vi "CANShark_SetBitrate.vi"(8 "Data Bitrate":i32, 9 "Nominal Bitrate":i32, 10 "Device Handler":i64, 11 "error in (no error)":errorcluster) -> (2 "CanFD Bitrate":u8, 3 "error out":errorcluster)   [LabVIEW 2026]
uses:
  x64/Release/CanSharkApi_Dll1.dll
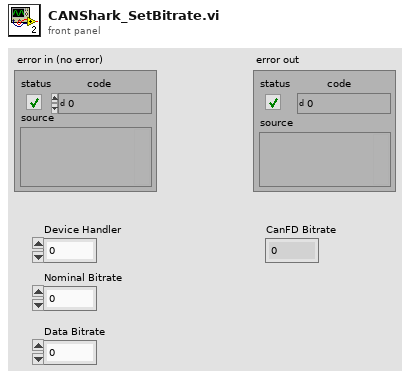
[diagram p1: front panel]
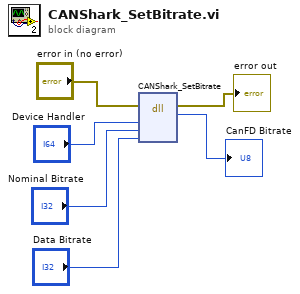
[diagram p0: block diagram]
diagram:
  n1 = dll-call lib="C:/Users/TECQNIO/Documents/CANSHARK LABVIEW API PACKAGE/x64/Release/CanSharkApi_Dll1.dll" fn="CANShark_SetBitrate"(error in="error in (no error)", "Device"="Device Handler", "nominal_bitrate"="Nominal Bitrate", "data_bitrate"="Data Bitrate") -> (error out=→"error out":errorcluster, "return type"=→"CanFD Bitrate":u8)  [unwired: 5 in, 1 out]
